vi "Operation.vi"(8 "error in (no error)":errorcluster, 11 "Arithemetic Operation in":refnum<class "Arithemetic Operation.lvclass">) -> (0 "error out":errorcluster, 2 "C":dbl, 3 "Arithemetic Operation out":refnum<class "Arithemetic Operation.lvclass">)   [LabVIEW 2023, in "Arithemetic Operation.lvclass"]
doc: "The VI is a method that performs the arithmetic operation and overrides the child classes methods."
uses:
  Arithemetic Operation.lvclass
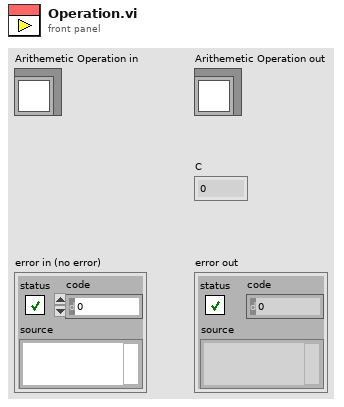
[diagram p1: front panel]
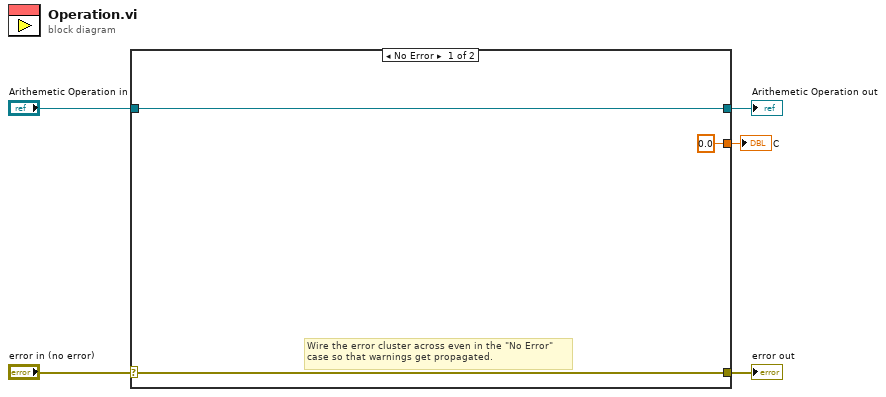
[diagram p0: block diagram]
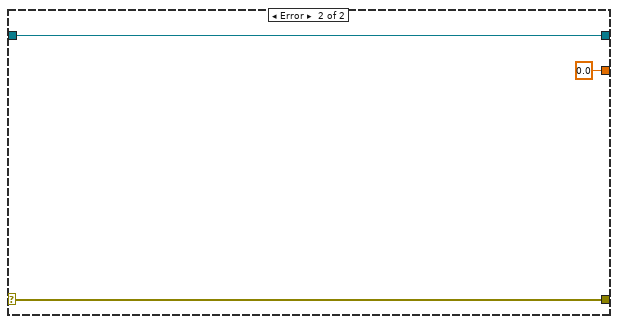
[diagram p2: hidden frame]
diagram:
  n1 = case shown="No Error" "error in (no error)" {
    selector: "error in (no error)" -> [w8 w11]
    tunnel: [w8 w11] -> w4
    tunnel: [w7 w10] -> w2
    tunnel: "Arithemetic Operation in" -> [w7 w10]
    tunnel: [0.0 0.0] -> w1
    frame No Error {
      # "Wire the error cluster across even in the \"No Error\"\ncase so that warnings get propagated."
    }
    frame Error {
    }
  }
  "error out" <- w4
  "Arithemetic Operation out" <- w2
  "C" <- w1
